vi "状态判断.vi"(8 "error IO":errorcluster, 9 "退出？":bool, 10 "簇 输入":cluster{"Data":string[], "State":T1}, 11 "队列输入":refnum<queue>) -> (2 "簇":cluster{"Data":string[], "State":T1})   [LabVIEW 2014]
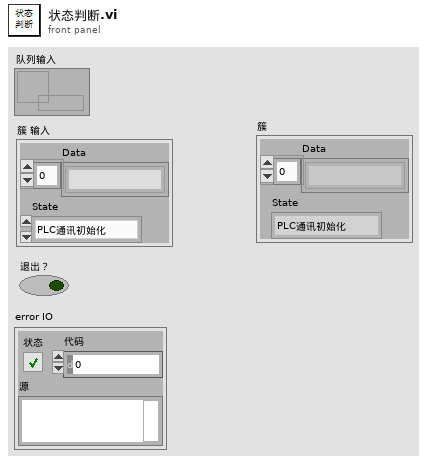
[diagram p1: front panel]
types:
  T1 = typedef "状态1.ctl" = enum16{"PLC通讯初始化", "---------------", "读左扫码请求", "读左二维码", "10左扫码回复", "--------------", "读扫码请求", "读二维码", "扫码回复", "-------------", "读数据保存请求", "读数据", "数据保存回复", "-----------------", "错误", "退出", "-------------------", "读扫码请求2", "读二维码2", "扫码回复2", "-- --------------", "读数据保存请求2", "读数据2", "数据保存回复2", "------------", "读扫码请求3", "读二维码3", "扫码回复3", "- ---------", "读数据保存请求3", "读数据3", "数据保存回复3", "----------", "看门狗", "------  --", "读料号请求1", "读料号1", "回复料号请求1", "--- ---- -", "读料号请求2", "读料号2", "回复料号请求2", "---- --------", "读料号请求3", "读料号3", "回复料号请求3", "-- - -  ------", "读料号请求4", "读料号4", "回复料号请求4", "---------- ---", "读PartNumber请求1", "读PartNumber1", "回复PartNumber请求1", "---------- ------", "读PartNumber请求2", "读PartNumber2", "回复PartNumber请求2", "---- -------------", "读PartNumber请求3", "读PartNumber3", "回复PartNumber请求3", "----------- ------", "读PartNumber请求4", "读PartNumber4", "回复PartNumber请求4"}
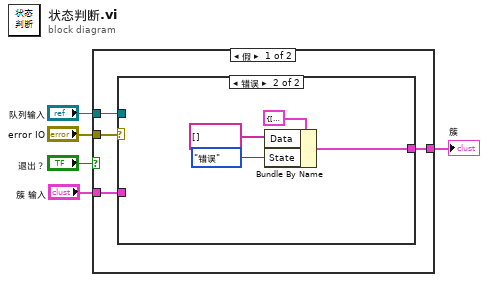
[diagram p0: block diagram]
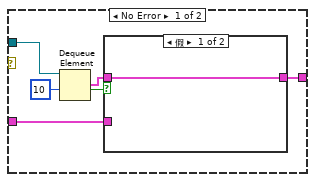
[diagram p2: hidden frame]
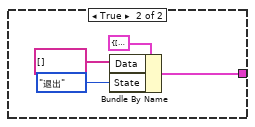
[diagram p4: hidden frame]
diagram:
  n1 = case shown="假" "退出？" {
    tunnel: "error IO" -> [w9 _]
    tunnel: "队列输入" -> [w8 _]
    tunnel: [w7 w22] -> w2
    tunnel: "簇 输入" -> [w6 _]
    frame False {
      n2 = case shown="错误" w9 {
        tunnel: w8 -> [w15 _]
        tunnel: [w11 w18] -> w7
        tunnel: w6 -> [w10 _]
        frame No Error {
          n3 = Dequeue Element(queue=w15, timeout in ms (-1)=10 ("超时毫秒(-1)")) -> (element=w12:cluster{"Data":string[], "State":T1}, timed out?=w13:bool)  [unwired: 1 in, 2 out]
          n4 = case shown="假" w13 {
            tunnel: w12 -> [w16 _]
            tunnel: [w16 w17] -> w11
            tunnel: w10 -> [_ w17]
            frame False {
            }
            frame True {
            }
          }
        }
        frame Error {
          n5 = Bundle By Name(cluster=cluster{"Data":string[], "State":T1} {"Data"=[], "State"=enum."PLC通讯初始化"} ("簇"), "Data"=string[] [], "State"=状态1."错误" ("PLC状态")) -> (w18:cluster{"Data":string[], "State":T1})
        }
      }
    }
    frame True {
      n6 = Bundle By Name(cluster=cluster{"Data":string[], "State":T1} {"Data"=[], "State"=enum."PLC通讯初始化"} ("簇"), "Data"=string[] [], "State"=状态1."退出" ("PLC状态")) -> (w22:cluster{"Data":string[], "State":T1})
    }
  }
  "簇" <- w2
